vi "Untitled 4.vi"(5 "Stop (F)":bool, 7 "error in":errorcluster) -> (20 "Image Out":T1(plugin-control), 26 "Stopped":bool, 27 "error out":errorcluster)   [LabVIEW 2017]
doc: "Creates, and edits acquisitions using the NI Vision Acquisition Express VI.\n\nThe NI Vision Acquisition Wizard is launched by placing the Express VI on the block diagram. Select an acquisition source and configure an acquisition using NI-IMAQ, NI-IMAQdx, or simulate an acquisition by reading an AVI or image files from a folder. After an acquisition is configured, select controls and indicators to be able to programmatically set in LabVIEW. Double-click the Vision Acquisition Express VI to edit the acquisition.\n\nNote: Any images created by the Express VI need to be disposed after use. Use the IMAQ Dispose.vi to cleanup the images output by the Express VI when they are no longer needed."
uses:
  <vilib>/vision/driver/NI_Vision_Acquisition_Software.lvlib
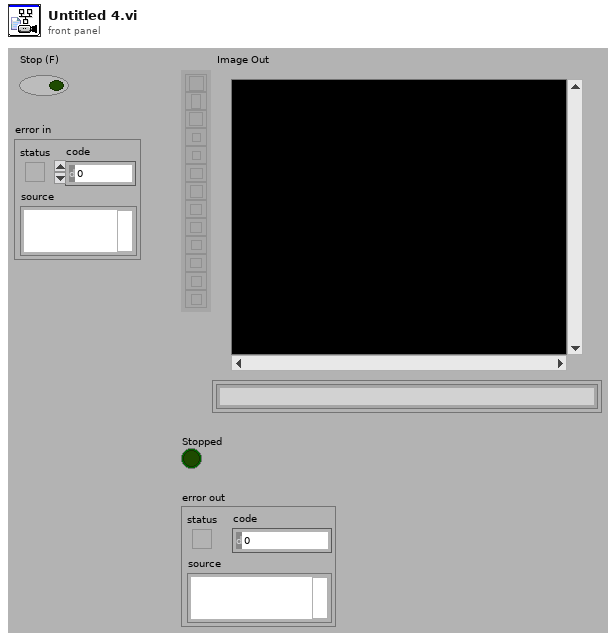
[diagram p1: front panel]
types:
  T1 = typedef "IMAQ Image.ctl" = refnum<image>
  T2 = typedef "IMAQdx.ctl" = refnum<k21>
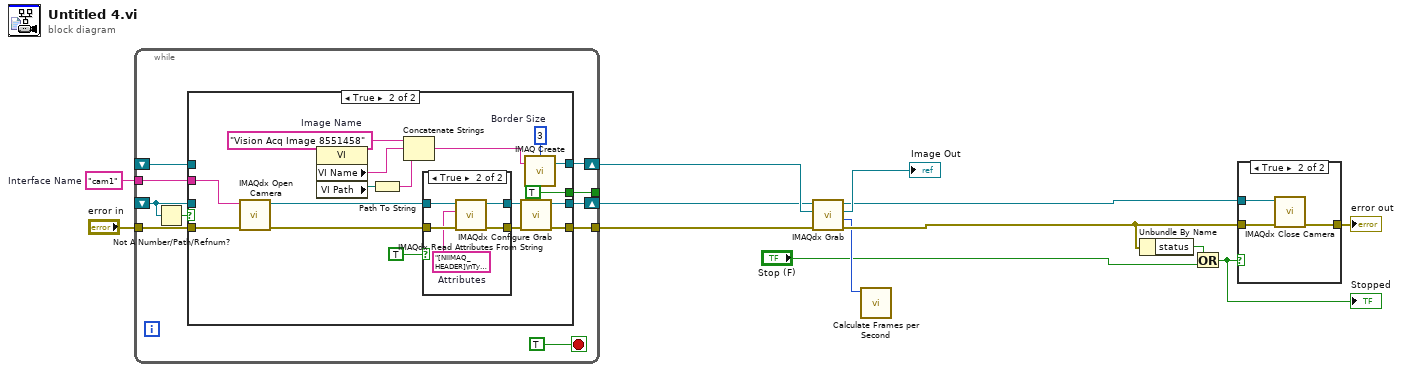
[diagram p0: block diagram]
diagram:
  w11 = "cam1"  # Interface Name
  n1 = while "While Loop_template0" {
    shift-right: [w23] -> w8
    shift-left: _ -> [w16]
    tunnel: [w22] -> w12
    tunnel: "error in" -> [w21]
    shift-right: [w19] -> w9
    shift-left: _ -> [w18]
    tunnel: w11 -> [w17]
    tunnel: [w14] -> _
    stop <- TRUE ("_template0") stop-if-true
    n2 = Not A Number/Path/Refnum?(number/path/refnum=w16) -> (NaN/Path/Refnum?=w15:bool)
    n3 = case "Case Structure_template0" shown="True" w15 {
      tunnel: [w26 w42] -> w23
      tunnel: w16 -> [w26 _]
      tunnel: [w25 w41] -> w22
      tunnel: w21 -> [w25 w43]
      tunnel: [w24 w40] -> w19
      tunnel: w18 -> [w24 _]
      tunnel: w17 -> [_ w30]
      tunnel: [_ TRUE] -> w14
      frame False {
      }
      frame True {
        w27 = 3  # Border Size
        w35 = "Vision Acq Image 8551458"  # Image Name
        n4 = call <vilib>:"IMAQdx Open Camera.vi"("error in"=w43, "Session In"=w30) -> ("error out"=w33:errorcluster, "Session Out"=w34:T2)  [unwired: 1 in, 7 out]
        n5 = property class="VI"() -> ("VI Name"=w38:string, "VI Path"=w39:path)  [unwired: 2 in, 2 out]
        n6 = Path To String(path=w39) -> (string=w37:string)
        n7 = Concatenate Strings(w35, w38, w37) -> (w36:string)
        n8 = case shown="True" TRUE ("Init Attributes") {
          tunnel: w34 -> [w45 w50]
          tunnel: w33 -> [w44 w49]
          tunnel: [w45 w47] -> w32
          tunnel: [w44 w46] -> w31
          frame False {
          }
          frame True {
            w48 = "[NIIMAQ_HEADER]\nType = 2\nVersion = 8\n\n[CAMERA_DATA]\nAcquisitionAttributes::Bayer::Algorithm = \"Bilinear\"\nAcquisitionAttributes::Bayer::GainB = \"1\"\nAcquisitionAttributes::Bayer::GainG = \"1\"\nAcquisitionAttributes::Bayer::GainR = \"1\"\nAcquisitionAttributes::Bayer::Pattern = \"Use hardware value\"\nAcquisitionAttributes::BitsPerPixel = \"Use hardware value\"\nAcquisitionAttributes::IgnoreFirstFrame = \"false\"\nAcquisitionAttributes::ImageDecoderCopyMode = \"Auto\"\nAcquisitionAttributes::OutputImageType = \"Auto\"\nAcquisitionAttributes::OverwriteMode = \"Get Newest\"\nAcquisitionAttributes::PixelSignedness = \"Use hardware value\"\nAcquisitionAttributes::ReceiveTimestampMode = \"None\"\nAcquisitionAttributes::ShiftPixelBits = \"false\"\nAcquisitionAttributes::SwapPixelBytes = \"false\"\nAcquisitionAttributes::Timeout = \"5000\"\nAcquisitionAttributes::VideoMode = \"640 x 480 YUY 2 30.00 fps\"\nCameraAttributes::BacklightCompensation::Mode = \"Manual\"\nCameraAttributes::BacklightCompensation::Value = \"1\"\nCameraAttributes::Brightness::Mode = \"Manual\"\nCameraAttributes::Brightness::Value = \"128\"\nCameraAttributes::Contrast::Mode = \"Manual\"\nCameraAttributes::Contrast::Value = \"32\"\nCameraAttributes::Exposure::Mode = \"Manual\"\nCameraAttributes::Exposure::Value = \"332\"\nCameraAttributes::Focus::Mode = \"Auto\"\nCameraAttributes::Gain::Mode = \"Manual\"\nCameraAttributes::Gain::Value = \"64\"\nCameraAttributes::Pan::Mode = \"Manual\"\nCameraAttributes::Pan::Value = \"0\"\nCameraAttributes::PowerLineFrequency::Mode = \"60Hz\"\nCameraAttributes::Saturation::Mode = \"Manual\"\nCameraAttributes::Saturation::Value = \"32\"\nCameraAttributes::Sharpness::Mode = \"Manual\"\nCameraAttributes::Sharpness::Value = \"22\"\nCameraAttributes::Tilt::Mode = \"Manual\"\nCameraAttributes::Tilt::Value = \"0\"\nCameraAttributes::WhiteBalance::Mode = \"Auto\"\nCameraAttributes::Zoom::Mode = \"Manual\"\nCameraAttributes::Zoom::Value = \"1\"\n"  # Attributes
            n9 = call <vilib>:"IMAQdx Read Attributes From String.vi"("error in"=w49, "Attributes String In"=w48, "Session In"=w50) -> ("error out"=w46:errorcluster, "Session Out"=w47:T2)  [unwired: 7 out]
          }
        }
        n10 = call <vilib>:"IMAQdx Configure Grab.vi"("error in"=w31, "Session In"=w32) -> ("error out"=w41:errorcluster, "Session Out"=w42:T2)  [unwired: 8 out]
        n11 = call "IMAQ Create"("Border Size"=w27, "Image Name"=w36) -> ("New Image"=w40:T1)  [unwired: 2 in, 2 out]
      }
    }
  }
  n12 = call <vilib>:"IMAQdx Grab.vi"("error in"=w12, "Image In"=w9, "Session In"=w8) -> ("error out"=w7:errorcluster, "Buffer Number Out"=w6:u32, "Image Out"=→"Image Out":T1, "Session Out"=w5:T2)  [unwired: 1 in, 4 out]
  n13 = call <vilib>:"Calculate Frames per Second.vi"("Buffer Number"=w6) -> ()  [unwired: 2 in, 9 out]
  n14 = Unbundle By Name(w7) -> ("status"=w1:bool)
  n15 = Or(x=w1, y="Stop (F)") -> (x .or. y?=w2:bool)
  "Stopped" <- w2
  n16 = case "Case Structure_template1" shown="True" w2 {
    tunnel: [w51 w53] -> w4
    tunnel: w7 -> [w51 w54]
    tunnel: w5 -> [_ w52]
    frame False {
    }
    frame True {
      n17 = call <vilib>:"IMAQdx Close Camera.vi"("error in"=w54, "Session In"=w52) -> ("error out"=w53:errorcluster)  [unwired: 9 out]
    }
  }
  "error out" <- w4
